vi "LifetimeHistogram.vi"(0 "1w Lifetime":dbl[][](array[numeric]), 1 "DC&1w Lifetime":dbl[][](array[numeric]), 2 "1w reference":refnum<vi>, 3 "DC&1w reference":refnum<vi>, 4 "Max Lifetime (s)":dbl=4e-09, 5 "Min Lifetime (s)":dbl=1e-09, 6 "Data Size":i32, 7 "error in (no error)":errorcluster, 8 "Bins":i32=1000) -> (13 "error out":errorcluster, 14 "1w Lifetime Hist":T1(graph)={"X Values"=array[1000 elements], "Histogram: h(x)"=[13, 27, 13, 19, 32, 22, 15, 16, 16, 16, 27, 21, 25, 18, 27, 21, 28, 22, 34, 24, 28, 18, 33, 20, 27, 26, 27, 35, 17, 17, 25, 33, 24, 20, 14, 23, 24, 30, 31, 35, 36, 32, 29, 19, 23, 24, 22, 23, 22, 25, 31, 29, 24, 36, 32, 25, 22, 34, 30, 39, 30, 33, 34, 23, 23, 32, 31, 32, 25, 28, 53, 27, 40, 37, 36, 42, 35, 26, 32, 36, 44, 53, 29, 28, 45, 37, 50, 37, 35, 35, 35, 33, 44, 50, 40, 42, 41, 41, 36, 41, 40, 37, 51, 51, 55, 61, 32, 37, 66, 54, 44, 46, 41, 42, 51, 52, 53, 40, 46, 50, 53, 49, 52, 57, 46, 51, 57, 60, 51, 60, 48, 46, 54, 62, 47, 56, 58, 59, 47, 40, 62, 54, 61, 68, 62, 78, 68, 74, 84, 66, 70, 64, 68, 71, 77, 78, 62, 64, 61, 95, 87, 79, 71, 85, 76, 62, 69, 69, 83, 67, 73, 87, 71, 86, 91, 87, 101, 82, 83, 90, 101, 107, 84, 90, 90, 94, 114, 100, 99, 107, 100, 88, 109, 93, 104, 106, 126, 128, 120, 129, 117, 112, 130, 126, 140, 127, 130, 151, 131, 124, 138, 138, 186, 151, 149, 152, 175, 152, 154, 164, 162, 149, 161, 164, 175, 156, 185, 170, 169, 199, 191, 215, 214, 184, 187, 201, 207, 206, 219, 264, 235, 237, 242, 253, 258, 273, 287, 286, 268, 284, 278, 291, 293, 277, 312, 311, 361, 330, 342, 291, 363, 351, 342, 335, 346, 379, 400, 399, 395, 408, 397, 387, 434, 500, 425, 431, 481, 473, 506, 504, 459, 511, 518, 510, 540, 551, 511, 515, 590, 529, 609, 631, 587, 578, 607, 626, 625, 622, 643, 660, 636, 696, 623, 691, 708, 679, 754, 723, 723, 764, 733, 725, 784, 780, 795, 787, 842, 804, 837, 826, 826, 848, 884, 878, 840, 911, 890, 886, 850, 834, 905, 891, 923, 968, 928, 894, 881, 931, 847, 921, 934, 903, 895, 935, 938, 876, 851, 857, 909, 974, 892, 877, 827, 888, 909, 861, 842, 857, 830, 861, 807, 880, 846, 904, 785, 861, 780, 760, 783, 728, 761, 730, 714, 721, 701, 680, 677, 688, 658, 657, 636, 642, 588, 614, 609, 592, 600, 555, 603, 556, 536, 537, 538, 484, 525, 533, 483, 456, 476, 470, 432, 454, 435, 429, 477, 417, 404, 381, 368, 403, 398, 402, 378, 354, 367, 336, 339, 339, 327, 333, 263, 304, 296, 299, 294, 316, 247, 276, 251, 233, 267, 247, 239, 245, 217, 260, 230, 242, 212, 187, 223, 181, 208, 204, 189, 207, 196, 174, 191, 182, 167, 168, 178, 146, 170, 174, 154, 160, 161, 153, 156, 136, 131, 143, 152, 147, 120, 138, 124, 107, 120, 127, 110, 100, 93, 107, 94, 115, 99, 110, 88, 92, 98, 90, 90, 100, 101, 91, 77, 97, 84, 99, 87, 74, 73, 66, 84, 72, 86, 88, 63, 73, 85, 76, 74, 66, 67, 68, 69, 65, 63, 69, 49, 62, 54, 63, 52, 51, 49, 54, 60, 54, 50, 45, 55, 52, 60, 67, 53, 52, 47, 56, 48, 48, 36, 41, 44, 56, 51, 37, 39, 45, 36, 39, 41, 43, 45, 51, 47, 41, 36, 33, 36, 35, 29, 34, 50, 40, 28, 33, 34, 31, 22, 30, 29, 30, 42, 25, 30, 33, 39, 23, 33, 29, 33, 26, 32, 33, 29, 29, 32, 36, 29, 30, 34, 39, 29, 29, 28, 29, 29, 27, 30, 33, 23, 22, 31, 28, 28, 21, 22, 32, 21, 26, 22, 15, 29, 24, 16, 31, 27, 22, 26, 20, 32, 30, 21, 22, 26, 12, 26, 23, 23, 18, 17, 24, 22, 28, 20, 25, 28, 23, 17, 17, 20, 40, 24, 19, 29, 24, 19, 20, 19, 22, 19, 26, 16, 25, 22, 15, 19, 20, 20, 20, 16, 19, 24, 20, 27, 11, 26, 19, 14, 22, 26, 20, 15, 16, 28, 19, 24, 20, 20, 13, 17, 32, 22, 22, 19, 22, 23, 22, 21, 17, 19, 9, 17, 10, 19, 21, 12, 18, 16, 12, 20, 16, 18, 15, 15, 12, 20, 13, 25, 17, 17, 20, 18, 11, 15, 20, 18, 18, 12, 19, 25, 16, 15, 16, 20, 16, 12, 17, 18, 19, 16, 8, 16, 16, 15, 15, 6, 18, 13, 14, 18, 17, 10, 21, 18, 13, 13, 12, 12, 18, 13, 22, 16, 19, 14, 23, 10, 14, 15, 10, 18, 7, 17, 9, 17, 14, 17, 13, 11, 6, 19, 15, 14, 11, 10, 10, 11, 9, 10, 11, 10, 23, 13, 15, 9, 12, 11, 10, 15, 15, 13, 12, 12, 13, 7, 10, 9, 10, 15, 4, 13, 8, 12, 10, 9, 7, 12, 11, 13, 10, 7, 10, 9, 11, 13, 9, 7, 11, 13, 11, 10, 12, 14, 6, 12, 10, 7, 13, 8, 8, 12, 8, 12, 15, 9, 15, 6, 14, 9, 12, 6, 9, 9, 10, 10, 5, 12, 6, 10, 11, 12, 7, 7, 11, 10, 18, 8, 5, 4, 11, 10, 9, 6, 5, 10, 10, 5, 6, 9, 8, 11, 5, 11, 10, 5, 5, 8, 14, 7, 5, 12, 7, 9, 7, 8, 2, 8, 11, 9, 4, 10, 7, 6, 7, 6, 6, 7, 3, 9, 4, 10, 11, 4, 5, 10, 6, 10, 3, 8, 8, 9, 8, 7, 9, 3, 6, 7, 6, 3, 11, 9, 7, 5, 8, 6, 9, 10, 9, 8, 5, 8, 9, 4, 5, 7, 2, 8, 3, 4, 4, 6, 7, 7, 4, 4, 5, 8, 4, 4, 7, 5, 8, 7, 6, 6, 7, 4, 5, 7, 1, 5, 8, 5, 9, 3, 4, 6, 6, 8, 9, 4, 4, 5, 7, 7, 8, 4, 3, 4, 7, 9, 7, 4, 5, 6, 3, 7, 5, 7, 2, 3, 5, 3, 5, 2, 2, 3, 3, 11, 0, 5, 4, 0, 9, 4, 7]}, 15 "DC&1w Lifetime Hist":T1(graph)={"X Values"=array[1000 elements], "Histogram: h(x)"=[1, 1, 1, 1, 3, 1, 4, 1, 0, 0, 0, 1, 1, 1, 2, 1, 4, 1, 2, 2, 1, 4, 2, 2, 2, 1, 0, 0, 2, 1, 4, 1, 0, 3, 1, 0, 4, 1, 2, 1, 1, 0, 1, 2, 0, 1, 2, 2, 2, 0, 1, 4, 0, 1, 1, 2, 0, 0, 1, 1, 1, 0, 3, 2, 0, 1, 3, 1, 4, 2, 2, 2, 1, 0, 2, 2, 2, 1, 2, 1, 4, 0, 2, 1, 3, 1, 1, 0, 1, 1, 0, 4, 3, 2, 2, 2, 2, 2, 0, 0, 0, 2, 2, 2, 1, 1, 2, 3, 2, 0, 1, 2, 2, 2, 2, 2, 0, 1, 0, 0, 3, 4, 3, 2, 0, 1, 0, 0, 1, 1, 3, 2, 1, 2, 3, 2, 2, 0, 1, 3, 1, 1, 3, 2, 1, 2, 3, 2, 0, 0, 2, 4, 2, 4, 0, 2, 1, 1, 2, 0, 1, 1, 1, 1, 0, 2, 1, 3, 0, 1, 1, 5, 7, 4, 3, 2, 2, 3, 1, 3, 2, 6, 3, 4, 1, 3, 0, 0, 2, 4, 3, 2, 2, 3, 3, 3, 5, 6, 7, 3, 2, 0, 1, 4, 8, 4, 0, 5, 4, 4, 0, 3, 4, 1, 3, 4, 4, 3, 8, 3, 3, 6, 4, 3, 6, 3, 3, 5, 2, 5, 3, 3, 4, 3, 2, 5, 3, 4, 5, 0, 7, 3, 6, 4, 7, 4, 8, 6, 5, 5, 3, 4, 6, 4, 3, 4, 4, 4, 6, 4, 5, 12, 2, 7, 4, 3, 7, 4, 5, 8, 3, 4, 2, 5, 9, 2, 10, 8, 12, 3, 3, 7, 10, 6, 10, 8, 3, 5, 7, 7, 8, 9, 10, 10, 5, 13, 13, 11, 9, 13, 15, 4, 6, 8, 9, 8, 6, 9, 21, 15, 7, 13, 6, 15, 11, 14, 12, 13, 20, 19, 14, 22, 26, 12, 16, 24, 21, 22, 30, 26, 24, 14, 26, 24, 27, 27, 44, 35, 38, 34, 55, 29, 51, 48, 56, 54, 69, 53, 55, 71, 65, 80, 84, 93, 81, 99, 79, 117, 119, 119, 123, 122, 141, 142, 152, 152, 148, 175, 155, 185, 194, 208, 210, 222, 222, 259, 265, 257, 233, 318, 276, 277, 318, 324, 340, 340, 344, 393, 389, 409, 460, 422, 408, 446, 440, 423, 456, 490, 475, 501, 479, 495, 500, 509, 508, 530, 503, 545, 563, 520, 555, 533, 589, 577, 567, 618, 585, 600, 588, 579, 617, 548, 599, 584, 577, 632, 597, 671, 623, 646, 602, 605, 617, 625, 604, 688, 638, 618, 639, 679, 632, 659, 673, 620, 660, 682, 623, 642, 684, 629, 649, 721, 639, 691, 639, 651, 645, 652, 637, 643, 673, 654, 650, 662, 651, 669, 641, 644, 619, 583, 638, 648, 622, 627, 627, 638, 647, 642, 574, 618, 588, 607, 569, 639, 593, 586, 606, 576, 559, 600, 580, 563, 584, 581, 560, 521, 565, 497, 544, 550, 542, 490, 534, 547, 503, 511, 498, 465, 480, 504, 468, 472, 484, 498, 528, 451, 513, 468, 506, 451, 447, 428, 454, 471, 453, 452, 451, 410, 448, 437, 439, 405, 411, 411, 398, 416, 413, 400, 397, 368, 367, 365, 371, 379, 363, 352, 373, 342, 365, 359, 383, 332, 369, 338, 356, 337, 341, 327, 306, 323, 324, 327, 281, 290, 310, 288, 282, 299, 288, 279, 281, 290, 247, 310, 263, 278, 292, 264, 293, 241, 244, 245, 277, 257, 254, 272, 267, 238, 273, 228, 232, 261, 219, 237, 240, 222, 216, 250, 223, 227, 241, 192, 221, 222, 220, 210, 233, 218, 182, 194, 190, 204, 228, 188, 173, 214, 197, 174, 187, 177, 204, 213, 187, 190, 191, 187, 204, 162, 179, 169, 177, 183, 161, 155, 168, 144, 177, 167, 169, 172, 163, 189, 157, 159, 138, 166, 176, 145, 160, 142, 153, 133, 170, 129, 144, 122, 131, 150, 126, 129, 145, 127, 141, 103, 127, 124, 122, 128, 119, 127, 114, 113, 115, 108, 132, 117, 122, 121, 118, 94, 123, 124, 112, 101, 124, 104, 90, 107, 111, 106, 113, 104, 105, 102, 98, 89, 99, 109, 109, 95, 97, 87, 106, 81, 109, 108, 107, 102, 89, 86, 81, 89, 88, 84, 83, 92, 90, 85, 90, 86, 97, 92, 73, 75, 87, 76, 73, 89, 80, 73, 78, 75, 59, 80, 74, 63, 86, 87, 71, 77, 66, 73, 72, 78, 85, 70, 81, 84, 70, 72, 81, 65, 71, 82, 57, 70, 65, 69, 60, 77, 71, 70, 71, 88, 69, 60, 71, 55, 66, 71, 71, 54, 59, 62, 61, 64, 65, 58, 63, 66, 64, 52, 64, 70, 56, 70, 72, 52, 51, 60, 66, 59, 59, 44, 54, 53, 49, 61, 47, 47, 35, 60, 51, 52, 48, 49, 54, 49, 50, 48, 40, 48, 47, 55, 55, 43, 41, 54, 36, 46, 51, 46, 39, 51, 42, 53, 50, 55, 41, 46, 59, 42, 44, 48, 42, 43, 45, 48, 27, 51, 40, 46, 45, 48, 46, 46, 43, 47, 48, 46, 30, 33, 43, 34, 48, 50, 39, 33, 44, 51, 26, 49, 46, 41, 37, 41, 42, 42, 47, 43, 39, 39, 39, 40, 35, 36, 41, 33, 35, 31, 43, 37, 36, 41, 26, 35, 35, 23, 36, 29, 38, 35, 38, 28, 33, 43, 38, 25, 34, 34, 40, 38, 33, 31, 32, 27, 35, 36, 28, 33, 36, 35, 37, 34, 30, 34, 25, 27, 28, 26, 35, 30, 37, 30, 28, 23, 30, 36, 17, 28, 28, 23, 25, 26, 36, 37, 33, 23, 31, 31, 22, 35, 25, 27, 24, 32, 25, 27, 25, 27, 24, 35, 26, 33, 20, 30, 15, 23, 29, 23, 30, 33, 32, 22, 20, 35, 27, 22, 28, 21, 22, 18, 20, 23, 22, 16, 22, 18, 34, 20, 26, 28, 25, 10, 20, 27, 26, 30, 19, 18, 25, 21, 21, 24, 28, 22, 23, 23, 22, 22]}, 16 "1w mean":dbl format="%.4g", 17 "1w std":dbl format="%.4g", 18 "DC&1w mean":dbl format="%.4g", 19 "DC&1w std":dbl format="%.4g")   [LabVIEW 2015]
uses:
  <vilib>/Analysis/NI_AALPro.lvlib
  <vilib>/Analysis/NI_AALBase.lvlib
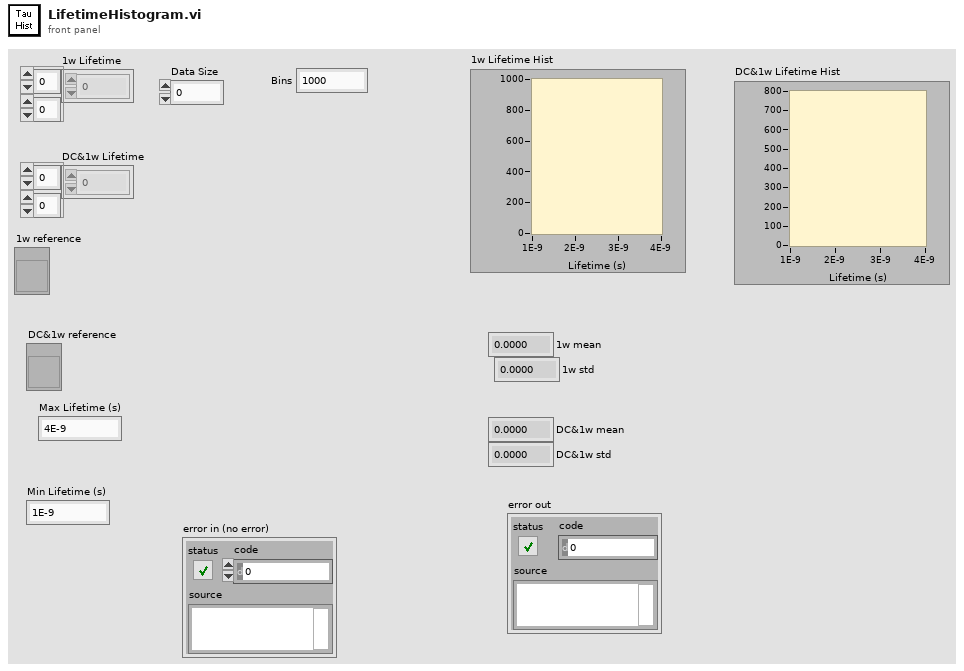
[diagram p1: front panel]
types:
  T1 = cluster{"X Values":dbl[], "Histogram: h(x)":i32[]}
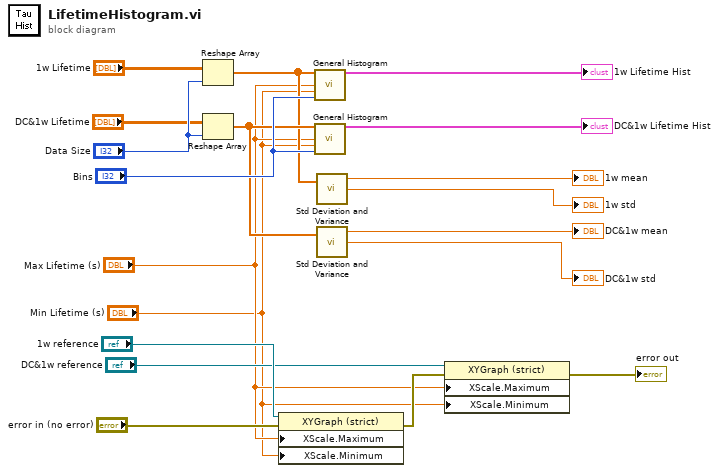
[diagram p0: block diagram]
diagram:
  n1 = Reshape Array("1w Lifetime", "Data Size") -> (w10:dbl[])
  n2 = Reshape Array("DC&1w Lifetime", "Data Size") -> (w13:dbl[])
  n3 = property class="XYGraph (strict)"(reference="1w reference", error in="error in (no error)", "XScale.Maximum"="Max Lifetime (s)", "XScale.Minimum"="Min Lifetime (s)") -> (error out=w4:errorcluster)  [unwired: 1 out]
  n4 = call <vilib>:"General Histogram.vi"("X"=w10, "max"="Max Lifetime (s)", "min"="Min Lifetime (s)", "# bins"="Bins") -> ("Histogram Graph"=→"1w Lifetime Hist":T1)  [unwired: 7 in, 4 out]
  n5 = call <vilib>:"General Histogram.vi"("X"=w13, "max"="Max Lifetime (s)", "min"="Min Lifetime (s)", "# bins"="Bins") -> ("Histogram Graph"=→"DC&1w Lifetime Hist":T1)  [unwired: 7 in, 4 out]
  n6 = call <vilib>:"Std Deviation and Variance.vi"("X"=w10) -> ("mean"=→"1w mean":dbl, "standard deviation"=→"1w std":dbl)  [unwired: 1 in, 1 out]
  n7 = call <vilib>:"Std Deviation and Variance.vi"("X"=w13) -> ("mean"=→"DC&1w mean":dbl, "standard deviation"=→"DC&1w std":dbl)  [unwired: 1 in, 1 out]
  n8 = property class="XYGraph (strict)"(reference="DC&1w reference", error in=w4, "XScale.Maximum"="Max Lifetime (s)", "XScale.Minimum"="Min Lifetime (s)") -> (error out=→"error out":errorcluster)  [unwired: 1 out]
